vi "philosopher.vi"(5 "Maximum attempts":i32, 6 "Maximum think time":u32=1000, 7 "Maximum eat time":u32=1000, 9 "total":i32, 10 "Ph id":i32) -> ()   [LabVIEW 2015]
uses:
  SINGLE_CHOP_Separator_string.ctl
panel:
  # "LOUNCHED FROM PHILOSOFERS"
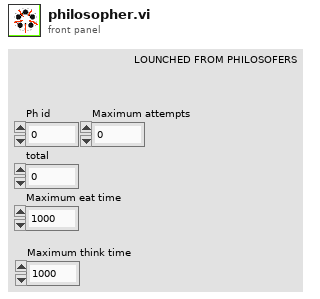
[diagram p1: front panel]
types:
  T1 = typedef "SINGLE_CHOP_Separator_string.ctl" = string
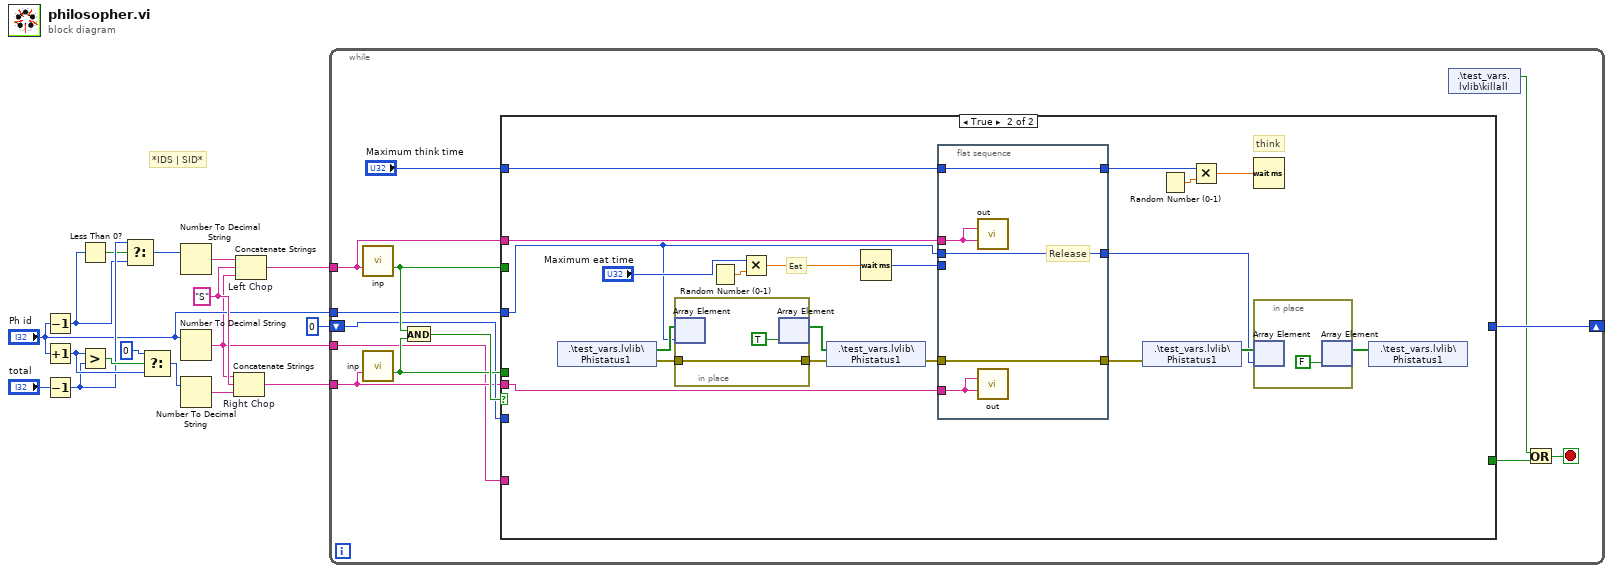
[diagram p0: block diagram]
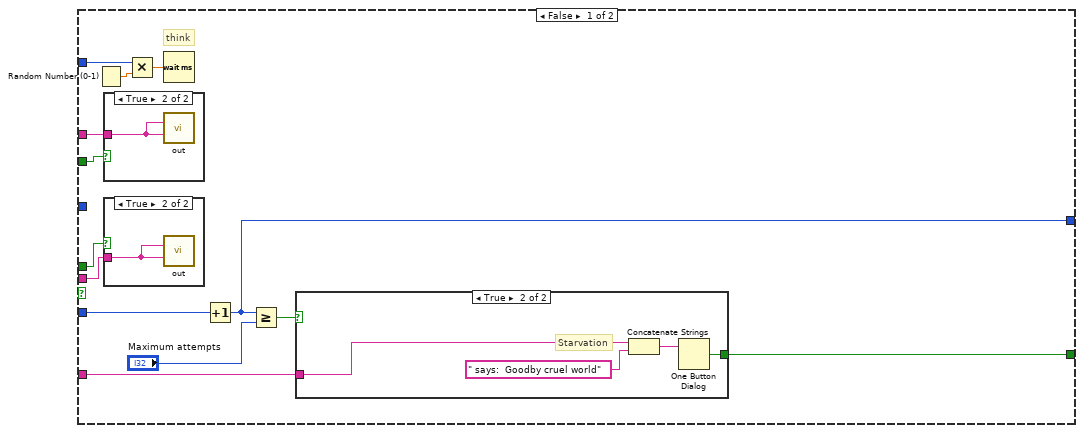
[diagram p2: hidden frame]
diagram:
  w9 = T1 "S"
  # "*IDS | SID*"
  n1 = Decrement(x="Ph id") -> (x-1=w7:i32)
  n2 = Increment(x="Ph id") -> (x+1=w14:i32)
  n3 = Decrement(x="total") -> (x-1=w12:i32)
  n4 = Less Than 0?(x=w7) -> (x < 0?=w6:bool)
  n5 = Greater?(x=w14, y=w12) -> (0:w13:bool)
  n6 = Select(t=w12, s=w6, f=w7) -> (s? t:f=w8:i32)
  n7 = Select(t=0, s=w13, f=w14) -> (s? t:f=w16:i32)
  n8 = Number To Decimal String(number=w8) -> (decimal integer string=w11:string)  [unwired: 1 in]
  n9 = Number To Decimal String(number="Ph id") -> (decimal integer string=w1:string)  [unwired: 1 in]
  n10 = Number To Decimal String(number=w16) -> (decimal integer string=w10:string)  [unwired: 1 in]
  n11 = Concatenate Strings "Right Chop"(w1, w9, w10) -> (w4:string)
  n12 = Concatenate Strings "Left Chop"(w11, w9, w1) -> (w5:string)
  n13 = while {
    shift-right: [w26] -> _
    shift-left: 0 -> [w27]
    tunnel: "Ph id" -> [w19]
    tunnel: w5 -> [w21]
    tunnel: w4 -> [w20]
    tunnel: w1 -> [w18]
    stop <- w23 stop-if-true
    n14 = call "inp.vi"("Name in"=w21) -> ("Valid data"=w29:bool)  [unwired: 12 in, 2 out]
    n15 = call "inp.vi"("Name in"=w20) -> ("Valid data"=w28:bool)  [unwired: 12 in, 2 out]
    n16 = And(x=w29, y=w28) -> (x .and. y?=w30:bool)
    n17 = case shown="True" w30 {
      tunnel: w21 -> [w41 w69]
      tunnel: w20 -> [w40 w68]
      tunnel: w29 -> [w43 _]
      tunnel: w28 -> [w42 _]
      tunnel: w27 -> [w39 _]
      tunnel: [w36 _] -> w22
      tunnel: [w35 _] -> w26
      tunnel: w18 -> [w32 _]
      tunnel: "Maximum think time" -> [w31 w61]
      tunnel: w19 -> [_ w54]
      frame False {
        # "think"
        n18 = Random Number (0-1)() -> (number: 0 to 1=w34:dbl)
        n19 = case shown="True" w43 {
          tunnel: w41 -> [_ w49]
          frame False {
          }
          frame True {
            n20 = call "out.vi"("IN VARIANT"=w49, "Name in"=w49) -> ()  [unwired: 12 in, 2 out]
          }
        }
        n21 = case shown="True" w42 {
          tunnel: w40 -> [_ w48]
          frame False {
          }
          frame True {
            n22 = call "out.vi"("IN VARIANT"=w48, "Name in"=w48) -> ()  [unwired: 12 in, 2 out]
          }
        }
        n23 = Multiply(x=w31, y=w34) -> (x*y=w33:dbl)
        n24 = Wait (ms)(milliseconds to wait=w33) -> ()  [unwired: 1 out]
        n25 = Increment(x=w39) -> (x+1=w35:i32)
        n26 = Greater Or Equal?(x=w35, y="Maximum attempts") -> (x >= y?=w37:bool)
        n27 = case shown="True" w37 {
          tunnel: [_ w47] -> w36
          tunnel: w32 -> [_ w46]
          frame False {
          }
          frame True {
            # "Starvation"
            n28 = Concatenate Strings(w46, " says:  Goodby cruel world" ("message")) -> (w44:string)
            n29 = One Button Dialog(message=w44) -> (true=w47:bool)  [unwired: 1 in]
          }
        }
      }
      frame True {
        # "think"
        # "Eat"
        n30 = shared-variable ".\\test_vars.lvlib\\Phistatus1"() -> (w59:bool[], error out=w52:errorcluster)  [unwired: 1 in]
        n31 = in-place {
          in-place-border: w52 -> [w71]
          in-place-border: [w71] -> w51
          n32 = in-place-array #1(w59, w54) -> ()  [unwired: 1 out]
          n33 = in-place-array #1(TRUE ("element")) -> (w58:bool[])  [unwired: 1 out]
        }
        n34 = Random Number (0-1)() -> (number: 0 to 1=w66:dbl)
        n35 = Multiply(x="Maximum eat time", y=w66) -> (x*y=w64:dbl)
        n36 = shared-variable ".\\test_vars.lvlib\\Phistatus1"(w58, error in=w51) -> (error out=w57:errorcluster)
        n37 = Wait (ms)(milliseconds to wait=w64) -> (millisecond timer value=w67:u32)
        n38 = flat-sequence {
          tunnel: w69 -> [w74]
          tunnel: w68 -> [w73]
          tunnel: w67 -> [_]
          tunnel: [w77] -> w60
          tunnel: w61 -> [w77]
          tunnel: w57 -> [w75]
          tunnel: [w76] -> w53
          tunnel: w54 -> [w76]
          tunnel: [w75] -> w50
          frame #0 {
            # "Release"
            n39 = call "out.vi"("IN VARIANT"=w74, "Name in"=w74) -> ()  [unwired: 12 in, 2 out]
            n40 = call "out.vi"("IN VARIANT"=w73, "Name in"=w73) -> ()  [unwired: 12 in, 2 out]
          }
        }
        n41 = shared-variable ".\\test_vars.lvlib\\Phistatus1"(error in=w50) -> (w55:bool[])  [unwired: 1 out]
        n42 = Random Number (0-1)() -> (number: 0 to 1=w63:dbl)
        n43 = Multiply(x=w60, y=w63) -> (x*y=w62:dbl)
        n44 = Wait (ms)(milliseconds to wait=w62) -> ()  [unwired: 1 out]
        n45 = in-place {
          n46 = in-place-array #2(w55, w53) -> ()  [unwired: 1 out]
          n47 = in-place-array #2(FALSE ("element")) -> (w56:bool[])  [unwired: 1 out]
        }
        n48 = shared-variable ".\\test_vars.lvlib\\Phistatus1"(w56) -> ()  [unwired: 1 in, 1 out]
      }
    }
    n49 = shared-variable ".\\test_vars.lvlib\\killall"() -> (w24:bool)  [unwired: 1 in, 1 out]
    n50 = Or(x=w24, y=w22) -> (x .or. y?=w23:bool)
  }
